vi "Servo MSMT GSM Configure DPD.vi"(8 "error in (no error)":errorcluster, 10 "Step In":refnum<k7>, 11 "Servo MSMT in":refnum<class "Servo MSMT.lvclass">) -> (0 "error out":errorcluster, 2 "Step Out":refnum<k7>, 3 "Servo MSMT out":refnum<class "Servo MSMT.lvclass">)   [LabVIEW 2018, in "Servo MSMT.lvlib" / "Servo MSMT.lvclass"]
uses:
  Servo MSMT.lvclass
  Plugins/TestStand API Tools (TSAT).lvlibp/Step Actions/TSAT Step Actions.lvlib
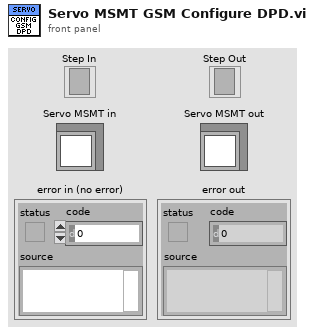
[diagram p1: front panel]
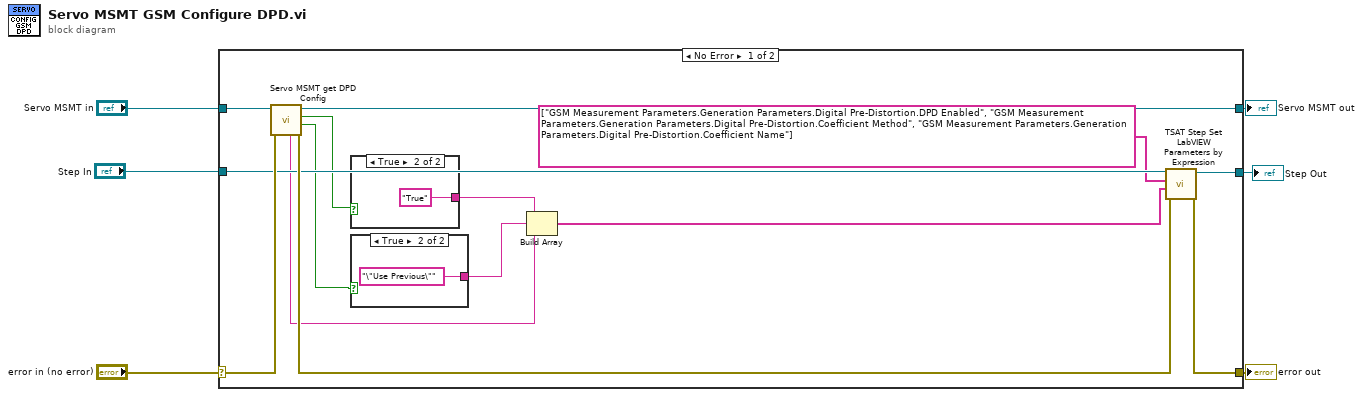
[diagram p0: block diagram]
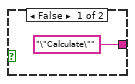
[diagram p2: hidden frame]
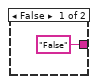
[diagram p3: hidden frame]
diagram:
  n1 = case shown="No Error" "error in (no error)" {
    selector: "error in (no error)" -> [w20 w27]
    tunnel: [w16 w27] -> w5
    tunnel: [w18 w26] -> w3
    tunnel: "Servo MSMT in" -> [w19 w26]
    tunnel: "Step In" -> [w15 w25]
    tunnel: [w14 w25] -> w1
    frame No Error {
      n2 = call "Servo MSMT get DPD Config.vi"("error in (no error)"=w20, "Servo MSMT in"=w19) -> ("error out"=w17:errorcluster, "USE LUT?"=w12:bool, "DPD Enabled?"=w13:bool, "Servo MSMT out"=w18:refnum<class "Servo MSMT.lvclass">, "LUT"=w9:string)  [unwired: 5 in]
      n3 = case shown="True" w13 {
        tunnel: ["False" "True"] -> w11
        frame False {
        }
        frame True {
        }
      }
      n4 = case shown="True" w12 {
        tunnel: ["\"Calculate\"" "\"Use Previous\""] -> w10
        frame False {
        }
        frame True {
        }
      }
      n5 = Build Array(w11, w10, w9) -> (w8:string[])
      n6 = call "TSAT Step Set LabVIEW Parameters by Expression.vi"("Error In"=w17, "Value Expressions"=w8, "Parameters to Set"=string[] ["GSM Measurement Parameters.Generation Parameters.Digital Pre-Distortion.DPD Enabled", "GSM Measurement Parameters.Generation Parameters.Digital Pre-Distortion.Coefficient Method", "GSM Measurement Parameters.Generation Parameters.Digital Pre-Distortion.Coefficient Name"], "Step In"=w15) -> ("Error Out"=w16:errorcluster, "Step Out"=w14:refnum<k7>)  [unwired: 6 in]
    }
    frame Error {
    }
  }
  "error out" <- w5
  "Servo MSMT out" <- w3
  "Step Out" <- w1
